vi "UpdateAzCamToolPanel.vi"(2 "Numeric Value":dbl, 3 "String Value":string, 4 "Control":T1(ring)) -> (0 "State":bool)   [LabVIEW 2014]
uses:
  globals/AzCamGlobals.vi
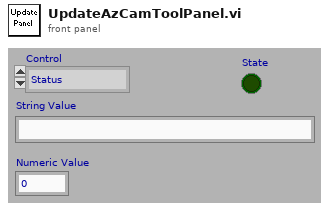
[diagram p1: front panel]
types:
  T1 = enum16{"Status", "CamTemp", "DewTemp", "GetExpose", "GetSequence", "SetExpose", "Filename", "ColBin", "RowBin"}
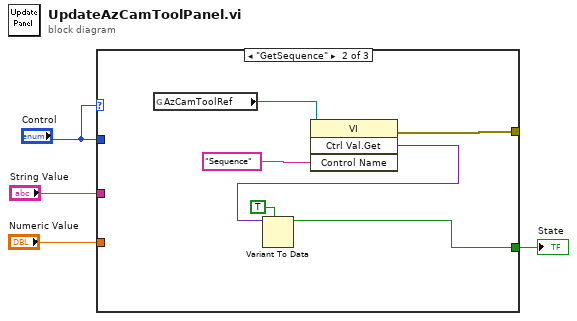
[diagram p0: block diagram]
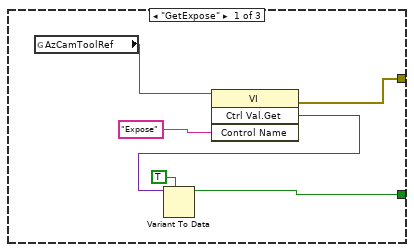
[diagram p2: hidden frame]
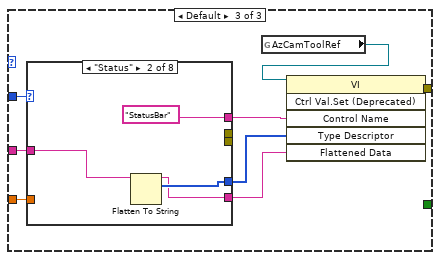
[diagram p3: hidden frame]
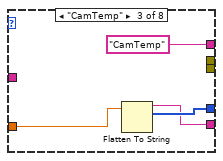
[diagram p5: hidden frame]
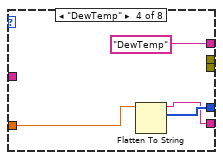
[diagram p6: hidden frame]
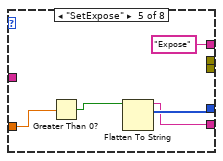
[diagram p7: hidden frame]
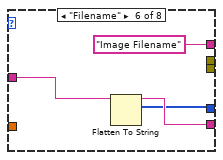
[diagram p8: hidden frame]
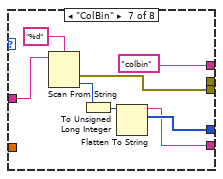
[diagram p9: hidden frame]
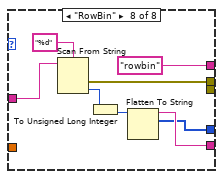
[diagram p10: hidden frame]
diagram:
  n1 = case shown="\"GetSequence\"" "Control" {
    tunnel: "Control" -> [_ _ w24]
    tunnel: "String Value" -> [_ _ w22]
    tunnel: [w7 w13 w19] -> _
    tunnel: "Numeric Value" -> [_ _ w18]
    tunnel: [w6 w12 _] -> w1
    frame "GetExpose" {
      n2 = global read "AzCamGlobals.vi" "AzCamToolRef"() -> (w5:refnum<vi>)
      n3 = invoke class="VI" method="Ctrl Val.Get"(reference=w5, "Control Name"="Expose") -> (error out=w7:errorcluster, "Get Control Value Variant"=w8:variant)  [unwired: 2 in, 2 out]
      n4 = Variant To Data(type=TRUE, Variant=w8) -> (data=w6:bool)  [unwired: 1 in, 1 out]
    }
    frame "GetSequence" {
      n5 = global read "AzCamGlobals.vi" "AzCamToolRef"() -> (w11:refnum<vi>)
      n6 = invoke class="VI" method="Ctrl Val.Get"(reference=w11, "Control Name"="Sequence") -> (error out=w13:errorcluster, "Get Control Value Variant"=w14:variant)  [unwired: 2 in, 2 out]
      n7 = Variant To Data(type=TRUE, Variant=w14) -> (data=w12:bool)  [unwired: 1 in, 1 out]
    }
    frame Default {
      n8 = case shown="\"Status\"" w24 {
        tunnel: [_ "StatusBar" ("Control Name") "CamTemp" ("Control Name") "DewTemp" ("Control Name") "Expose" ("Control Name") "Image Filename" ("Control Name") "colbin" ("Control Name") "rowbin" ("Control Name")] -> w23
        tunnel: w22 -> [_ w25 _ _ _ w42 w50 w56]
        tunnel: [_ w27 w31 w35 w40 w43 w52 w59] -> w21
        tunnel: [_ w26 w30 w34 w39 w44 w51 w60] -> w20
        tunnel: w18 -> [_ _ w29 w33 w41 _ _ _]
        tunnel: [_ _ _ _ _ _ w46 _] -> _
        tunnel: [_ _ _ _ _ _ _ w54] -> _
        frame Default {
        }
        frame "Status" {
          n9 = Flatten To String(anything=w25) -> (data string=w26:string, type string=w27:i16[])  [unwired: 3 in, 1 out]
        }
        frame "CamTemp" {
          n10 = Flatten To String(anything=w29) -> (data string=w30:string, type string=w31:i16[])  [unwired: 3 in, 1 out]
        }
        frame "DewTemp" {
          n11 = Flatten To String(anything=w33) -> (data string=w34:string, type string=w35:i16[])  [unwired: 3 in, 1 out]
        }
        frame "SetExpose" {
          n12 = Greater Than 0?(x=w41) -> (x > 0?=w38:bool)
          n13 = Flatten To String(anything=w38) -> (data string=w39:string, type string=w40:i16[])  [unwired: 3 in, 1 out]
        }
        frame "Filename" {
          n14 = Flatten To String(anything=w42) -> (data string=w44:string, type string=w43:i16[])  [unwired: 3 in, 1 out]
        }
        frame "ColBin" {
          n15 = Scan From String(format string="%d", input string=w50) -> (error out=w46:errorcluster, output 1=w49:i32)  [unwired: 3 in, 2 out]
          n16 = To Unsigned Long Integer(number=w49) -> (unsigned 32bit integer=w47:u32)
          n17 = Flatten To String(anything=w47) -> (data string=w51:string, type string=w52:i16[])  [unwired: 3 in, 1 out]
        }
        frame "RowBin" {
          n18 = Scan From String(format string="%d", input string=w56) -> (error out=w54:errorcluster, output 1=w57:i32)  [unwired: 3 in, 2 out]
          n19 = To Unsigned Long Integer(number=w57) -> (unsigned 32bit integer=w55:u32)
          n20 = Flatten To String(anything=w55) -> (data string=w60:string, type string=w59:i16[])  [unwired: 3 in, 1 out]
        }
      }
      n21 = global read "AzCamGlobals.vi" "AzCamToolRef"() -> (w17:refnum<vi>)
      n22 = invoke class="VI" method="Ctrl Val.Set (Deprecated)"(reference=w17, "Control Name"=w23, "Type Descriptor"=w21, "Flattened Data"=w20) -> (error out=w19:errorcluster)  [unwired: 2 in, 5 out]
    }
  }
  "State" <- w1
